vi "Tosca-Get Pretrial Property Table (MATLAB).vi"(0 "Path":path, 11 "error in (no error)":errorcluster) -> (8 "Table":T1[](array[typedef]), 15 "error out":errorcluster)   [LabVIEW 2020]
uses:
  epl-vi-lib/Utility VIs/Controls/KPropertyTable/RowData.ctl
  epl-vi-lib/Utility VIs/Controls/KPropertyTable/DataType.ctl
  <vilib>/regexp/Match Regular Expression.xnode
  epl-vi-lib/Utility VIs/Controls/KPropertyTable/KPropertyTable.xctl
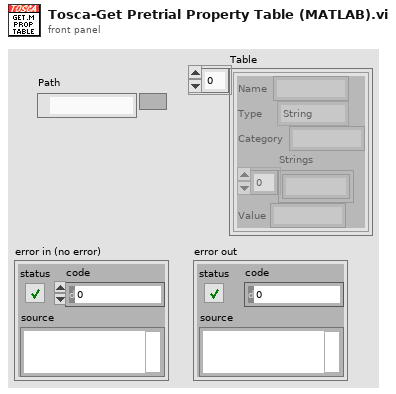
[diagram p1: front panel]
types:
  T1 = typedef "KPropertyTable.xctl/RowData.ctl" = cluster{"Name":string, "Type":T2, "Category":string, "Strings":string[], "Value":string}
  T2 = typedef "KPropertyTable.xctl/DataType.ctl" = enum16{"String", "Enum", "Int", "Double", "Boolean", "Ring", "Formula"}
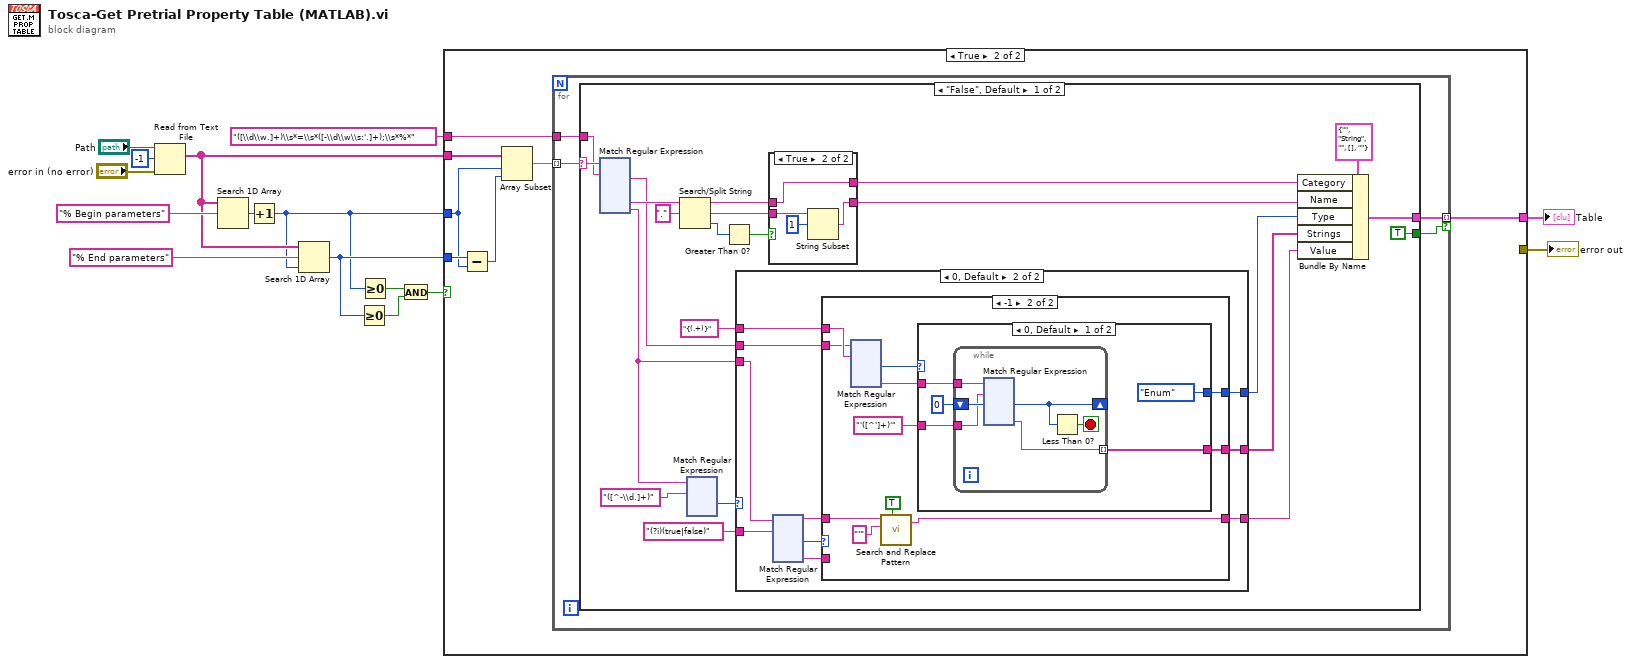
[diagram p0: block diagram]
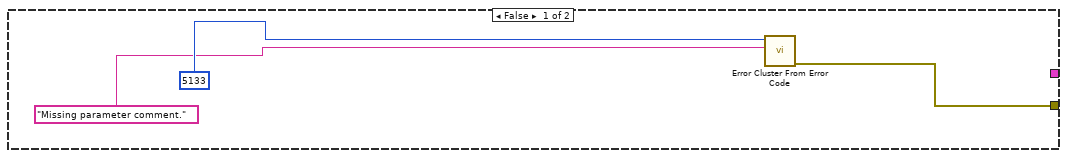
[diagram p2: hidden frame]
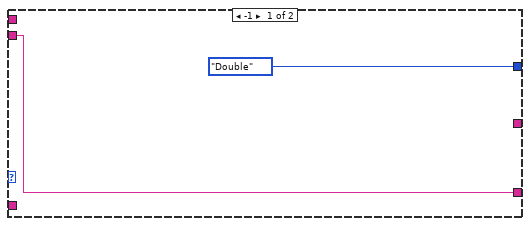
[diagram p3: hidden frame]
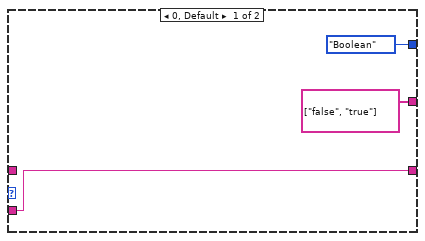
[diagram p4: hidden frame]
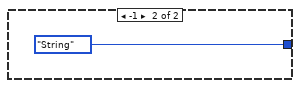
[diagram p5: hidden frame]
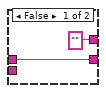
[diagram p6: hidden frame]
diagram:
  n1 = Read from Text File(file (use dialog)="Path", count=-1, error in="error in (no error)") -> (text=w5:string[])  [unwired: 1 in, 3 out]
  n2 = Search 1D Array(1D array=w5, element="% Begin parameters") -> (index of element=w8:i32)  [unwired: 1 in]
  n3 = Increment(x=w8) -> (x+1=w3:i32)
  n4 = Search 1D Array(1D array=w5, element="% End parameters", start index (0)=w3) -> (index of element=w9:i32)
  n5 = Greater Or Equal To 0?(x=w9) -> (x >= 0?=w11:bool)
  n6 = Greater Or Equal To 0?(x=w3) -> (x >= 0?=w12:bool)
  n7 = And(x=w12, y=w11) -> (x .and. y?=w10:bool)
  n8 = case shown="True" w10 {
    tunnel: w9 -> [_ w24]
    tunnel: w3 -> [_ w23]
    tunnel: w5 -> [_ w25]
    tunnel: [w16 _] -> w7
    tunnel: "([\\d\\w.]+)\\s*=\\s*([-\\d\\w\\s:'.]+);\\s*%*" -> [_ w20]
    tunnel: [_ w19] -> w1
    frame False {
      n9 = call <vilib>:"Error Cluster From Error Code.vi"("error message (\"\")"="Missing parameter comment.", "error code (0)"=5133) -> ("error out"=w16:errorcluster)  [unwired: 7 in]
    }
    frame True {
      n10 = Subtract(x=w24, y=w23) -> (x-y=w22:i32)
      n11 = Array Subset(array=w25, index=w23, length=w22) -> (w21:string[])
      n12 = for {
        tunnel: w21 -> [w29] mode=indexing
        tunnel: w20 -> [w28]
        tunnel: [w27] -> w19 mode=indexing if=w26
        n13 = case shown="\"False\", Default" w29 {
          selector: w29 -> [w51 _]
          tunnel: w28 -> [w50 _]
          tunnel: [w47 _] -> w27
          tunnel: [TRUE _] -> w26
          frame "False", Default {
            n14 = xnode "Match Regular Expression"("input string"=w51, "regular expression"=w50) -> ("after match"=w35:string, "submatch 1"=w45:string, "submatch 2"=w32:string)  [unwired: 4 in, 4 out]
            n15 = Search/Split String(string=w45, search string/char (-)=".") -> (substring before match=w42:string, match + rest of string=w39:string, offset of match=w44:i32)  [unwired: 1 in]
            n16 = xnode "Match Regular Expression"("input string"=w32, "regular expression"="([^-\\d.]+)") -> ("offset past match"=w33:i32)  [unwired: 4 in, 4 out]
            n17 = Greater Than 0?(x=w44) -> (x > 0?=w43:bool)
            n18 = case shown="0, Default" w33 {
              tunnel: [w52 w60] -> w37
              tunnel: [DataType."Double" ("Type") w59] -> w36
              tunnel: w35 -> [_ w55]
              tunnel: "(?i)(true|false)" ("regular expression") -> [_ w63]
              tunnel: w32 -> [w52 w57]
              tunnel: "{(.+)}" ("regular expression") -> [_ w56]
              tunnel: [_ w54] -> w30
              frame -1 {
              }
              frame 0, Default {
                n19 = xnode "Match Regular Expression"("input string"=w57, "regular expression"=w63) -> ("before match"=w58:string, "offset past match"=w62:i32, "submatch 1"=w61:string)  [unwired: 4 in, 3 out]
                n20 = case shown="-1" w62 {
                  tunnel: w61 -> [w66 _]
                  tunnel: [w66 w69] -> w60
                  tunnel: [DataType."Boolean" ("Type") w77] -> w59
                  tunnel: w58 -> [_ w70]
                  tunnel: w56 -> [_ w76]
                  tunnel: w55 -> [_ w73]
                  tunnel: [string[] ["false", "true"] w67] -> w54
                  frame 0, Default {
                  }
                  frame -1 {
                    n21 = xnode "Match Regular Expression"("input string"=w73, "regular expression"=w76) -> ("offset past match"=w75:i32, "submatch 1"=w74:string)  [unwired: 4 in, 4 out]
                    n22 = call <vilib>:"Search and Replace Pattern.vi"("string"=w70, "regular expression (\"\")"="'" ("regular expression (\"\")"), "replace all? (F)"=TRUE) -> ("result string"=w69:string)  [unwired: 2 in, 1 out]
                    n23 = case shown="0, Default" w75 {
                      tunnel: [DataType."Enum" ("Type") DataType."String" ("Type")] -> w77
                      tunnel: w74 -> [w81 _]
                      tunnel: "'([^']+)'" -> [w79 _]
                      tunnel: [w78 _] -> w67
                      frame 0, Default {
                        n24 = while {
                          tunnel: w81 -> [w87]
                          shift-right: [w86] -> _
                          shift-left: 0 -> [w88]
                          tunnel: w79 -> [w84]
                          tunnel: [w83] -> w78 mode=indexing
                          stop <- w85 stop-if-true
                          n25 = xnode "Match Regular Expression"("input string"=w87, "regular expression"=w84, "offset (0)"=w88) -> ("offset past match"=w86:i32, "submatch 1"=w83:string)  [unwired: 3 in, 4 out]
                          n26 = Less Than 0?(x=w86) -> (x < 0?=w85:bool)
                        }
                      }
                      frame -1 {
                      }
                    }
                  }
                }
              }
            }
            n27 = case shown="True" w43 {
              tunnel: w42 -> [w553 w557]
              tunnel: [w553 w555] -> w41
              tunnel: ["" w557] -> w40
              tunnel: w39 -> [_ w556]
              frame False {
              }
              frame True {
                n28 = String Subset(string=w556, offset (0)=1) -> (substring=w555:string)  [unwired: 1 in]
              }
            }
            n29 = Bundle By Name(cluster=T1 {"Name"="", "Type"=enum."String", "Category"="", "Strings"=[], "Value"=""} ("Row"), "Category"=w40, "Name"=w41, "Type"=w36, "Strings"=w30, "Value"=w37) -> (w47:T1)
          }
          frame "" {
          }
        }
      }
    }
  }
  "error out" <- w7
  "Table" <- w1
